vi "Generate Z stack Image File Names.vi"(8 "error in (no error)":errorcluster, 9 "Z Stack Image Folder Path":path, 10 "Z Stage Image Folder Name":string, 11 "Z Stack Size":i32) -> (0 "error out":errorcluster, 1 "Green Channel File Paths":path[](array[path]), 3 "Red Channel Image Names":string[](array[string]), 4 "Green Channel Image Names":string[](array[string]), 5 "Red Channel File Paths":path[](array[path]))   [LabVIEW 2020]
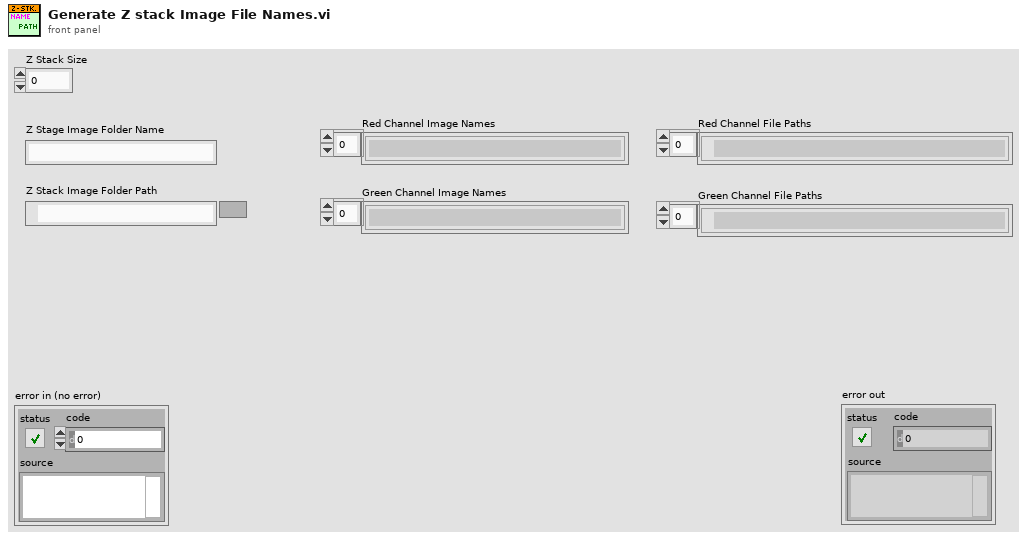
[diagram p1: front panel]
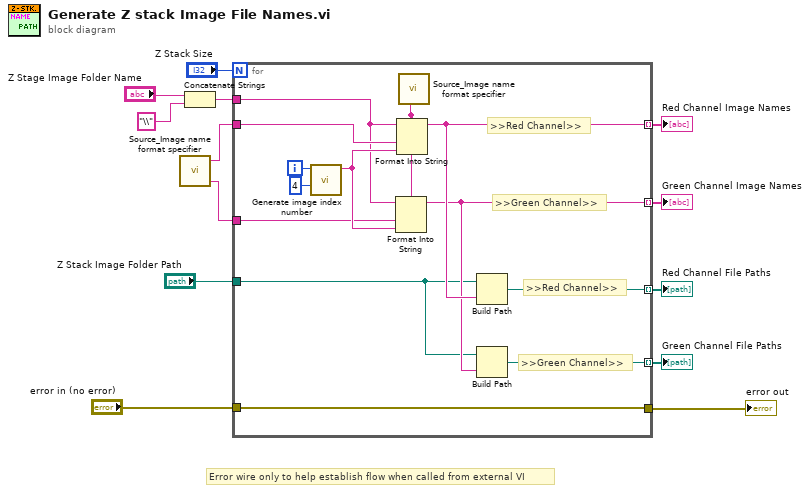
[diagram p0: block diagram]
diagram:
  # "Error wire only to help establish flow when called from external VI"
  n1 = call "Source_Image name format specifier.vi"() -> ("Red channel name"=w12:string, "Green channel name"=w11:string)  [unwired: 5 in, 1 out]
  n2 = Concatenate Strings("Z Stage Image Folder Name", "\\" ("string")) -> (w8:string)
  n3 = for {
    N: "Z Stack Size" -> [_]
    tunnel: w12 -> [w22]
    tunnel: w11 -> [w21]
    tunnel: w8 -> [w20]
    tunnel: [w19] -> w6 mode=indexing
    tunnel: [w17] -> w5 mode=indexing
    tunnel: "Z Stack Image Folder Path" -> [w16]
    tunnel: [w18] -> w4 mode=indexing
    tunnel: [w15] -> w3 mode=indexing
    tunnel: "error in (no error)" -> [w14]
    tunnel: [w14] -> w1
    i -> [w24]
    # ">>Green Channel>>"
    # ">>Red Channel>>"
    # ">>Green Channel>>"
    # ">>Red Channel>>"
    n4 = call "Generate image index number.vi"("Minimum Width (4)"=i16 4, "FOR loop iteration or existing number of files"=w24) -> ("Number in string representation (padded with zeroes)"=w25:string)  [unwired: 9 in]
    n5 = call "Source_Image name format specifier.vi"() -> ("Z-Stack Image name format specifier"=w26:string)  [unwired: 5 in, 2 out]
    n6 = Format Into String(format string=w26, initial string=w20, w21, w25) -> (resulting string=w17:string)  [unwired: 1 in, 1 out]
    n7 = Format Into String(format string=w26, initial string=w20, w22, w25) -> (resulting string=w19:string)  [unwired: 1 in, 1 out]
    n8 = Build Path(base path=w16, name or relative path=w19) -> (appended path=w18:path)
    n9 = Build Path(base path=w16, name or relative path=w17) -> (appended path=w15:path)
  }
  "Red Channel Image Names" <- w6
  "Green Channel Image Names" <- w5
  "Red Channel File Paths" <- w4
  "Green Channel File Paths" <- w3
  "error out" <- w1
